vi "CRYPolar Plot.vi"(4 "Pen":T1={"Width"=1, "Style"=enum."Solid"}, 5 "[user-specified font]":T4, 6 "polar attributes":T2={"maximum"=0.0, "minimum"=0.0, "clip to min"=FALSE, "log?(F)"=FALSE, "grid color"=6710886, "plot color"=65280, "fmt and prec"={"format"=enum."Decimal", "precision"=0}, "visible section"=8} {"minimum" format="%0.2f"; "maximum" format="%0.2f"}, 7 "desired font(Application)":T3(ring)=enum."Application Font", 8 "top left point(0, 0)":cluster{"x":i16, "y":i16}, 9 "dimensions (w,h)":cluster{"width":i16, "height":i16}, 10 "data array [mag, phase (deg)]":cluster{"magnitude":dbl, "phase":dbl}[](array[cluster]) {"phase" format="%0.2f"; "magnitude" format="%0.2f"}, 11 "picture":picture) -> (3 "new picture":picture)   [LabVIEW 2013]
doc: "Takes a picture and polar data and appends a picture that represents a polar graph of the data."
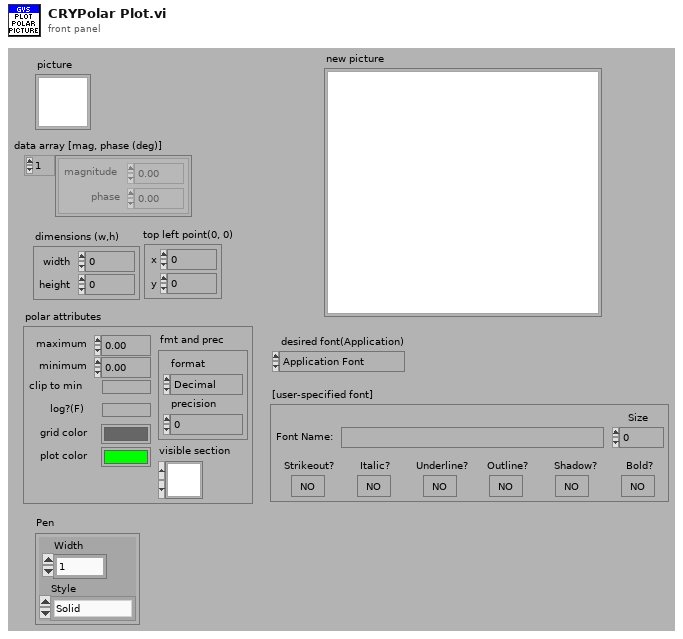
[diagram p1: front panel]
types:
  T1 = cluster{"Width":u16, "Style":enum32{"Solid", "Dash", "Dot", "DashDot", "DashDotDot"}}
  T2 = cluster{"maximum":dbl, "minimum":dbl, "clip to min":bool, "log?(F)":bool, "grid color":u32, "plot color":u32, "fmt and prec":cluster{"format":enum8{"Decimal", "Scientific", "Engineering", "Binary", "Octal", "Hex"}, "precision":u8}, "visible section":u16}
  T3 = enum16{"User-specified Font", "Application Font", "System Font", "Dialog Font"}
  T4 = cluster{"Font Name:":string, "Size":i16, "Strikeout?":bool, "Italic?":bool, "Underline?":bool, "Outline?":bool, "Shadow?":bool, "Bold?":bool}
  T5 = cluster{"left":i16, "top":i16, "right":i16, "bottom":i16}
  T6 = cluster{"pixel center":cluster{"x":i16, "y":i16}, "scale factors":cluster{"a":dbl, "b":dbl, "log?":bool}, "grid color":u32, "start angle":dbl, "end angle":dbl, "tick length":i16, "pixel radius":i32}
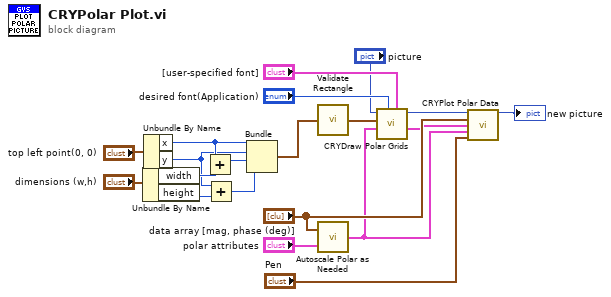
[diagram p0: block diagram]
diagram:
  n1 = Unbundle By Name("dimensions (w,h)") -> ("width"=w8:i16, "height"=w7:i16)
  n2 = Unbundle By Name("top left point(0, 0)") -> ("x"=w6:i16, "y"=w5:i16)
  n3 = Add(x=w6, y=w8) -> (x+y=w4:i16)
  n4 = Add(x=w5, y=w7) -> (x+y=w3:i16)
  n5 = Bundle("x"=w6, "y"=w5, w4, w3) -> (w2:cluster{"x":i16, "y":i16, i16, i16})  [unwired: 1 in]
  n6 = call <vilib>:"Validate Rectangle.vi"("rect"=w2) -> ("valid rect"=w11:T5)
  n7 = call <vilib>:"Autoscale Polar as Needed.vi"("polar attributes"="polar attributes", "data"="data array [mag, phase (deg)]") -> ("polar attributes"=w13:T2)
  n8 = call "CRYDraw Polar Grids.vi"("[user-specified font]"="[user-specified font]", "desired font(Application)"="desired font(Application)", "polar attributes"=w13, "rect"=w11, "picture"="picture") -> ("grid measurements"=w12:T6, "new picture"=w14:picture)  [unwired: 5 in]
  n9 = call "CRYPlot Polar Data.vi"("picture"=w14, "polar data"="data array [mag, phase (deg)]", "grid measurements"=w12, "polar attributes"=w13, "pen"="Pen") -> ("new picture"=→"new picture":picture)  [unwired: 10 in]
